vi "Strip EthernetFrame (IP).vi"(11 "IP Frame In":u8[](array[numeric]) format="%.0x") -> (2 "IP header":T1, 3 "IP Frame Out":u8[](array[numeric]) format="%.0x")   [LabVIEW 2020, in "EthFrameManagement.lvlib"]
uses:
  EthFrameManagement.lvlib
  controls/IPFrame_type.ctl
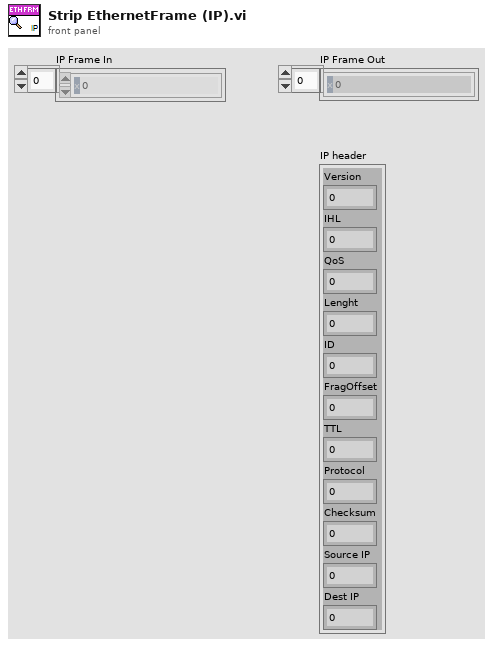
[diagram p1: front panel]
types:
  T1 = typedef "EthFrameManagement.lvlib/IPFrame_type.ctl" = cluster{"Version":u8, "IHL":u8, "QoS":u8, "Lenght":u16, "ID":u16, "FragOffset":u16, "TTL":u8, "Protocol":u8, "Checksum":u16, "Source IP":u32, "Dest IP":u32}
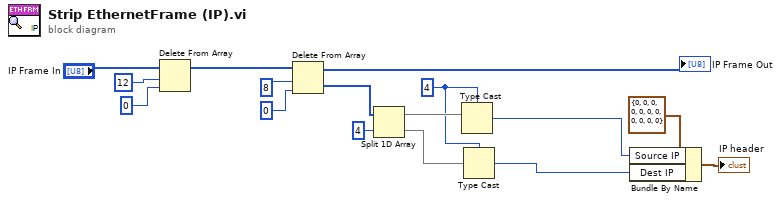
[diagram p0: block diagram]
diagram:
  w3 = u32 4 ("index")
  n1 = Delete From Array(array="IP Frame In", length=12, index=0) -> (array with subset deleted=w11:u8[])  [unwired: 1 out]
  n2 = Delete From Array(array=w11, length=8, index=0) -> (deleted portion=w7:u8[], array with subset deleted=→"IP Frame Out":u8[])
  n3 = Split 1D Array(array=w7, index=4) -> (first subarray=w5:u8[], second subarray=w4:u8[])
  n4 = Type Cast(type=w3, x=w5) -> (*(type *) &x=w2:u32)
  n5 = Type Cast(type=w3, x=w4) -> (*(type *) &x=w1:u32)
  n6 = Bundle By Name(cluster=T1 {"Version"=0, "IHL"=0, "QoS"=0, "Lenght"=0, "ID"=0, "FragOffset"=0, "TTL"=0, "Protocol"=0, "Checksum"=0, "Source IP"=0, "Dest IP"=0} ("IP Header"), "Source IP"=w2, "Dest IP"=w1) -> (→"IP header":T1)
